vi "p2 solution.vi"(11 "Dir List":cluster{"Name":string, "Size":i64}[](array[cluster])) -> (3 "Numeric":i64)   [LabVIEW 2021, in "d7.lvlib"]
uses:
  d7.lvlib
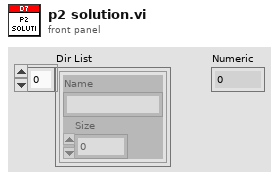
[diagram p1: front panel]
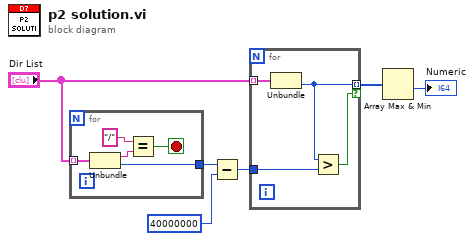
[diagram p0: block diagram]
diagram:
  n1 = for {
    tunnel: "Dir List" -> [w11] mode=indexing
    tunnel: [w8] -> w5
    stop <- w9 stop-if-true
    n2 = Unbundle(w11) -> ("Name"=w10:string, "Size"=w8:i64)
    n3 = Equal?(x="/", y=w10) -> (x = y?=w9:bool)
  }
  n4 = Subtract(x=w5, y=i64 40000000 ("Size")) -> (x-y=w6:i64)
  n5 = for {
    tunnel: "Dir List" -> [w12] mode=indexing
    tunnel: w6 -> [w15]
    tunnel: [w13] -> w3 mode=indexing if=w14
    n6 = Unbundle(w12) -> ("Size"=w13:i64)  [unwired: 1 out]
    n7 = Greater?(x=w13, y=w15) -> (0:w14:bool)
  }
  n8 = Array Max & Min(array=w3) -> (min value=→"Numeric":i64)  [unwired: 3 out]
